vi "New Analog Reader.vi"(8 "error in (no error)":errorcluster, 9 "Loop Period in ms (10)":u32=10, 10 "DAQmx Task":refnum<k21>, 11 "Analog Reader in":refnum<class "Analog Reader.lvclass">) -> (0 "error out":errorcluster, 3 "Analog Reader out":refnum<class "Analog Reader.lvclass">)   [LabVIEW 2024]
uses:
  Analog Reader.lvclass
  Analog Reader.lvclass/Analog Reader.ctl
  C:/Users/ottoa/OneDrive/Desktop/working copies/DAQmxActor/src/DAQmx Actor/DAQmx Actor/DAQmx Actor.lvclass
  C:/Program Files (x86)/National Instruments/LabVIEW 2024/vi.lib/ActorFramework/Actor/Actor.lvclass
  C:/Users/ottoa/OneDrive/Desktop/working copies/DAQmxActor/src/DAQmx Actor/Analog Reader/Analog Reader.lvclass
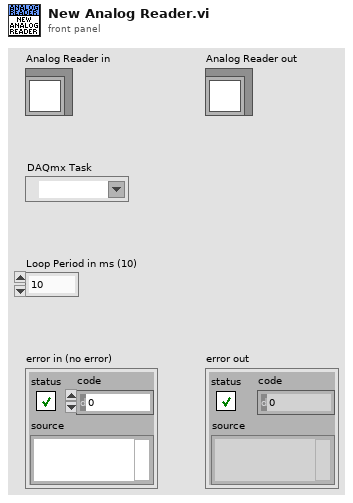
[diagram p1: front panel]
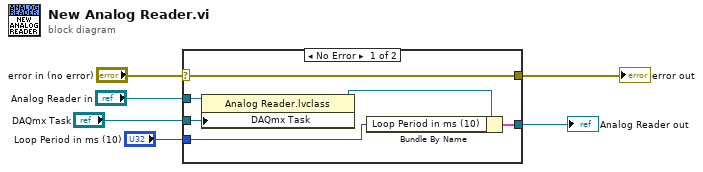
[diagram p0: block diagram]
diagram:
  n1 = case shown="No Error" "error in (no error)" {
    selector: "error in (no error)" -> [w12 w14]
    tunnel: [w12 w14] -> w5
    tunnel: [w9 w13] -> w3
    tunnel: "Analog Reader in" -> [w11 w13]
    tunnel: "DAQmx Task" -> [w8 _]
    tunnel: "Loop Period in ms (10)" -> [w7 _]
    frame No Error {
      n2 = property class="Analog Reader.lvclass"(reference=w11, "DAQmx Task"=w8) -> (reference out=w10:refnum<class "Analog Reader.lvclass">)  [unwired: 1 in, 1 out]
      n3 = Bundle By Name(cluster=w10, "Loop Period in ms (10)"=w7) -> (w9:cluster{})
    }
    frame Error {
    }
  }
  "error out" <- w5
  "Analog Reader out" <- w3
